vi "Event_GetRefAndReg.vi"(8 "error in":errorcluster) -> (0 "error out":errorcluster, 3 "Event Refnum":T1, 4 "Event Registration Refnum":T2)   [LabVIEW 2022 SP3, in "hse-misc.lvlib"]
doc: "Gets the HSE-Event refnum and a new event registration refnum for it.\n\n\n\n____\nHAMPEL SOFTWARE ENGINEERING v3.8.0 (2023-12-18 14:41)"
uses:
  hse-misc.lvlib
  Event_GenericRegistration.ctl
  Event_GenericReference.ctl
  Event_GenericDatatype.ctl
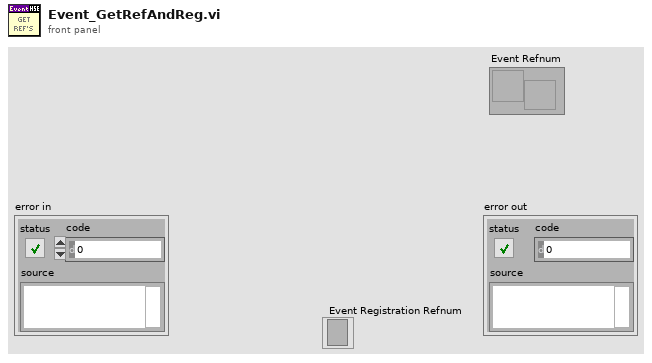
[diagram p1: front panel]
types:
  T1 = typedef "hse-misc.lvlib/Event_GenericReference.ctl" = refnum<user-event>
  T2 = typedef "hse-misc.lvlib/Event_GenericRegistration.ctl" = refnum<event-registration>
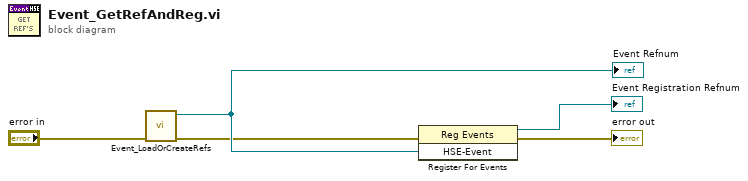
[diagram p0: block diagram]
diagram:
  n1 = call "Event_LoadOrCreateRefs.vi"("Error In"="error in") -> ("Error Out"=w2:errorcluster, "HSE-Event"=w4:T1)  [unwired: 9 in]
  "Event Refnum" <- w4
  n2 = register-events(error in=w2, w4) -> (reference out=→"Event Registration Refnum":refnum<event-registration>, error out=→"error out":errorcluster)  [unwired: 1 in]
